vi "process.vi"(8 "error in (no error)":errorcluster, 10 "Process":string, 11 "Processor in":refnum<class "Processor.lvclass">) -> (0 "error out":errorcluster, 2 "Variant":variant, 3 "Processor out":refnum<class "Processor.lvclass">)   [LabVIEW 2025, in "Processor.lvclass"]
uses:
  Processor.lvclass
  Processor.lvclass/Processor.ctl
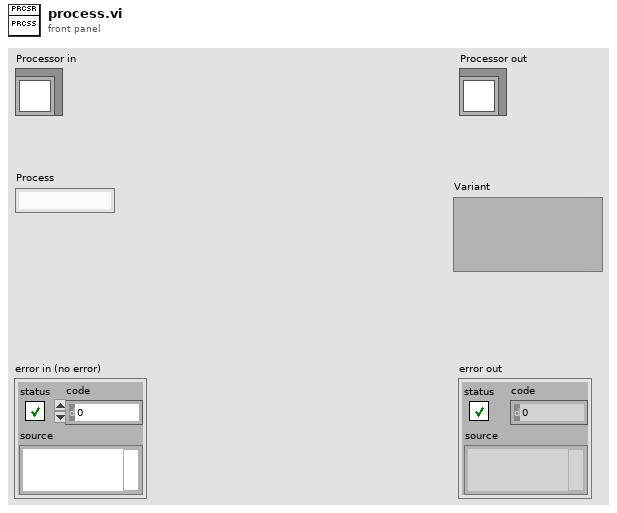
[diagram p1: front panel]
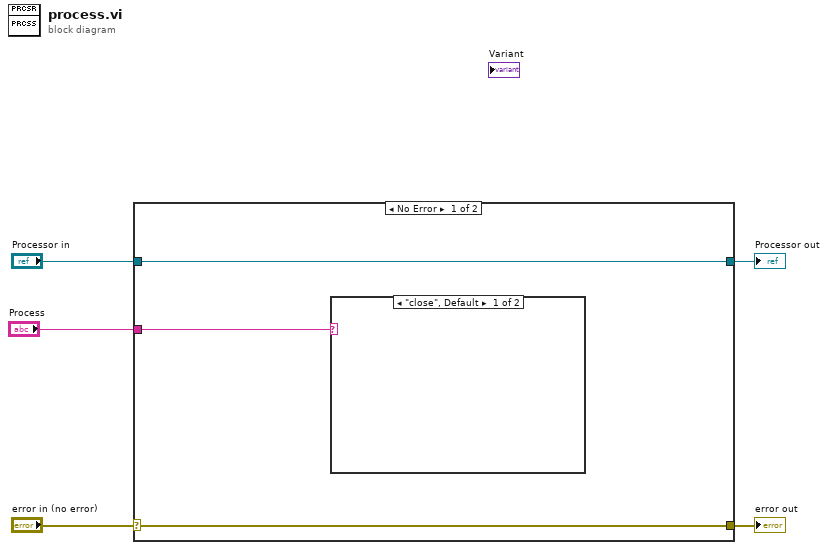
[diagram p0: block diagram]
diagram:
  n1 = case shown="No Error" "error in (no error)" {
    selector: "error in (no error)" -> [w7 w10]
    tunnel: [w7 w10] -> w4
    tunnel: [w8 w9] -> w2
    tunnel: "Processor in" -> [w8 w9]
    tunnel: "Process" -> [w6 _]
    frame No Error {
      n2 = case shown="\"close\", Default" w6 {
        frame "close", Default {
        }
        frame "init" {
        }
      }
    }
    frame Error {
    }
  }
  "error out" <- w4
  "Processor out" <- w2
